vi "Insert Paquete.vi"(8 "error in (no error)":errorcluster, 11 "Paquete":string) -> (0 "error out":errorcluster)   [LabVIEW 2020, in "Contabilidad.lvlib"]
uses:
  Contabilidad.lvlib
  <vilib>/drjdpowell/SQLite Library/SQL Connection/Open (path).vi
  <vilib>/drjdpowell/SQLite Library/SQL Connection/Open (string).vi
  <vilib>/AdvancedString/Path To Command Line String.vi
  <vilib>/drjdpowell/SQLite Library/SQL Connection/Execute SQL (No results).vi
  <vilib>/drjdpowell/SQLite Library/SQL Connection/Connection.lvclass
  <vilib>/drjdpowell/SQLite Library/SQLite.lvlib
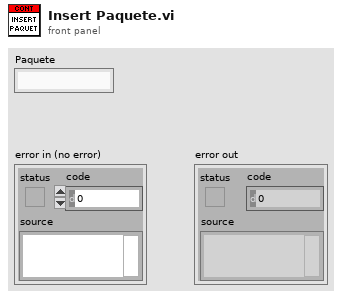
[diagram p1: front panel]
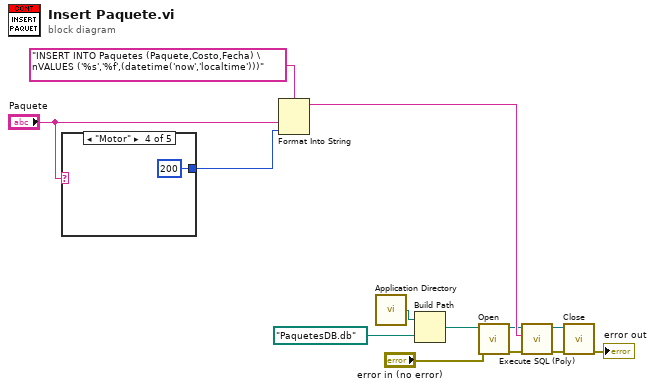
[diagram p0: block diagram]
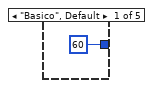
[diagram p2: hidden frame]
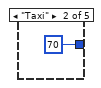
[diagram p3: hidden frame]
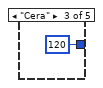
[diagram p4: hidden frame]
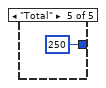
[diagram p5: hidden frame]
diagram:
  n1 = case shown="\"Motor\"" "Paquete" {
    tunnel: [60 70 120 200 250] -> w1
    frame "Basico", Default {
    }
    frame "Taxi" {
    }
    frame "Cera" {
    }
    frame "Motor" {
    }
    frame "Total" {
    }
  }
  n2 = Format Into String(format string="INSERT INTO Paquetes (Paquete,Costo,Fecha) \nVALUES ('%s','%f',(datetime('now','localtime')))", "Paquete", w1) -> (resulting string=w10:string)  [unwired: 2 in, 1 out]
  n3 = call <vilib>:"Application Directory.vi"() -> ("Application Directory"=w9:path)
  n4 = Build Path(base path=w9, name or relative path=path "PaquetesDB.db") -> (appended path=w7:path)
  n5 = call-poly <vilib>:"Open.vi"("error in (no error)"="error in (no error)", "db file"=w7) -> ("error out"=w12:errorcluster, "SQLite Connection"=w6:refnum<class "Connection.lvclass">)  [unwired: 8 in]
  n6 = call-poly <vilib>:"Execute SQL (Poly).vi"("error in (no error)"=w12, "SQL"=w10, "SQLite Connection in"=w6) -> ("error out"=w13:errorcluster, "SQLite Connection"=w5:refnum<class "Connection.lvclass">)  [unwired: 7 in]
  n7 = call-dynamic "Close.vi"("error in (no error)"=w13, "SQLite Connection in"=w5) -> ("error out"=→"error out":errorcluster)  [unwired: 9 in]
